vi "ATF-Storage-In Range.vi"(3 "Min":dbl format="%#_13g", 4 "X":dbl format="%#_13g", 5 "Max":dbl format="%#_13g") -> (1 "In Range":bool)   [LabVIEW 2022 SP3]
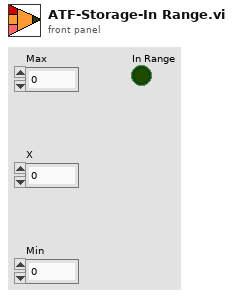
[diagram p1: front panel]
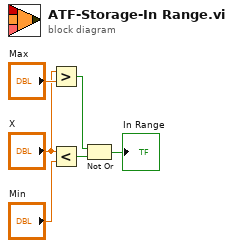
[diagram p0: block diagram]
diagram:
  n1 = Greater?(x="X", y="Max") -> (0:w5:bool)
  n2 = Less?(x="X", y="Min") -> (x < y?=w4:bool)
  n3 = Not Or(1:w4, 2:w5) -> (0:→"In Range":bool)
